vi "Optical Encoder Counter 2.vi"(9 "Input in":dbl, 10 "Last Value in":bool, 11 "Stopped":bool) -> (2 "Input out":dbl, 3 "Last Value out":bool)   [LabVIEW 2020]
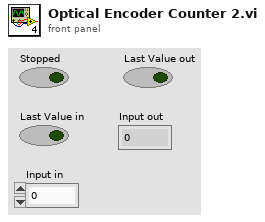
[diagram p1: front panel]
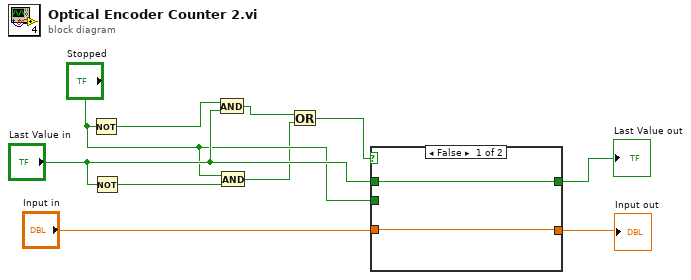
[diagram p0: block diagram]
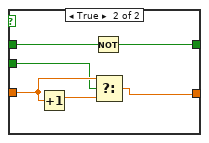
[diagram p2: hidden frame]
diagram:
  n1 = Not(x="Stopped") -> (.not. x?=w1:bool)
  n2 = Not(x="Last Value in") -> (.not. x?=w2:bool)
  n3 = And(x=w1, y="Last Value in") -> (x .and. y?=w4:bool)
  n4 = And(x="Stopped", y=w2) -> (x .and. y?=w3:bool)
  n5 = Or(x=w4, y=w3) -> (x .or. y?=w5:bool)
  n6 = case shown="False" w5 {
    tunnel: "Input in" -> [w11 w18]
    tunnel: "Stopped" -> [_ w16]
    tunnel: [w11 w15] -> w10
    tunnel: "Last Value in" -> [w12 w14]
    tunnel: [w12 w13] -> w8
    frame False {
    }
    frame True {
      n7 = Increment(x=w18) -> (x+1=w17:dbl)
      n8 = Not(x=w14) -> (.not. x?=w13:bool)
      n9 = Select(t=w18, s=w16, f=w17) -> (s? t:f=w15:dbl)
    }
  }
  "Input out" <- w10
  "Last Value out" <- w8
